vi "Mutate New CMD.vi"(0 "Class Library in":refnum<vi>, 1 "Line 2 text":string, 2 "Line 1 text":string, 5 "Command name":string, 7 "Wait For Response?":bool, 9 "Timeout":i32, 11 "error in":errorcluster) -> (4 "Class Library out":refnum<vi>, 15 "error out":errorcluster)   [LabVIEW 2012, in "REx_Springboard.lvlib"]
uses:
  REx_Springboard.lvlib
  <vilib>/LabVIEW Icon API/API_Text.ctl
  <vilib>/LabVIEW Icon API/API_Test Settings.ctl
  <vilib>/LabVIEW Icon API/lv_icon/Controls/Alignment.ctl
  <vilib>/LabVIEW Icon API/API_Text Colors.ctl
  <vilib>/LabVIEW Icon API/LabVIEW Icon API.lvlib
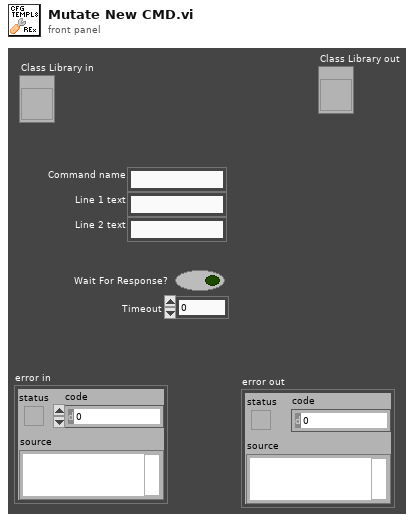
[diagram p1: front panel]
types:
  T1 = typedef "LabVIEW Icon API.lvlib/API_Text.ctl" = cluster{"Line 1 text":string, "Line 2 text":string, "Line 3 text":string, "Line 4 text":string}
  T2 = typedef "LabVIEW Icon API.lvlib/API_Test Settings.ctl" = cluster{"Font":string, "Alignment":T3, "Size":u8, "Center text":bool, "Capitalize text":bool, "Text color":T4}
  T3 = typedef "Alignment.ctl" = u16
  T4 = typedef "LabVIEW Icon API.lvlib/API_Text Colors.ctl" = cluster{"Line 1 color":u32, "Line 2 color":u32, "Line 3 color":u32, "Line 4 color":u32}
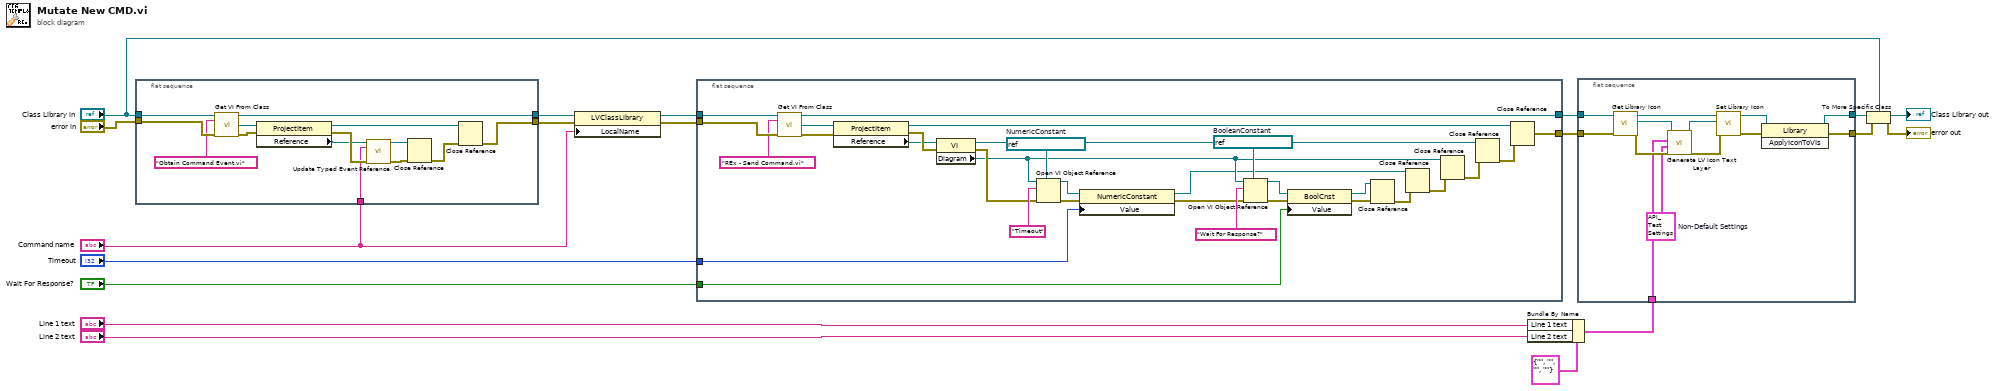
[diagram p0: block diagram]
diagram:
  n1 = flat-sequence {
    tunnel: [w27] -> w10
    tunnel: "Class Library in" -> [w26]
    tunnel: "error in" -> [w25]
    tunnel: [w20] -> w12
    tunnel: "Command name" -> [w23]
    frame #0 {
      n2 = call "Get VI From Class.vi"("Class Library"=w26, "Class Item Name"="Obtain Command Event.vi" ("Current Name 3"), "error in"=w25) -> ("Class Library"=w27:refnum<vi>, "Class Item Refnum"=w32:refnum<vi>, "error out"=w28:errorcluster)  [unwired: 10 in]
      n3 = property class="ProjectItem"(reference=w32, error in=w28) -> (reference out=w22:refnum<vi>, error out=w33:errorcluster, "Reference"=w31:refnum<vi>)
      n4 = call "Update Typed Event Reference.vi"("vi reference in"=w31, "Command Name"=w23, "error in"=w33) -> ("vi reference out"=w30:refnum<vi>, "error out"=w29:errorcluster)  [unwired: 11 in]
      n5 = Close Reference(reference=w30, error in (no error)=w29) -> (error out=w21:errorcluster)
      n6 = Close Reference(reference=w22, error in (no error)=w21) -> (error out=w20:errorcluster)
    }
  }
  n7 = property class="LVClassLibrary"(reference=w10, error in=w12, "LocalName"="Command name") -> (reference out=w13:refnum<vi>, error out=w15:errorcluster)
  n8 = flat-sequence {
    tunnel: "Wait For Response?" -> [w56]
    tunnel: [w34] -> w9
    tunnel: w13 -> [w55]
    tunnel: [w54] -> w14
    tunnel: w15 -> [w52]
    tunnel: "Timeout" -> [w49]
    frame #0 {
      w59 = refnum<vi> refnum  # BooleanConstant
      w61 = refnum<vi> refnum  # NumericConstant
      n9 = call "Get VI From Class.vi"("Class Library"=w55, "Class Item Name"="REx - Send Command.vi" ("name/order"), "error in"=w52) -> ("Class Library"=w54:refnum<vi>, "Class Item Refnum"=w53:refnum<vi>, "error out"=w46:errorcluster)  [unwired: 10 in]
      n10 = property class="ProjectItem"(reference=w53, error in=w46) -> (reference out=w44:refnum<vi>, error out=w64:errorcluster, "Reference"=w63:refnum<vi>)
      n11 = property class="VI"(reference=w63, error in=w64) -> (reference out=w43:refnum<vi>, error out=w50:errorcluster, "Diagram"=w42:refnum<vi>)
      n12 = Open VI Object Reference(7:w61, 8:w50, 10:"Timeout" ("name/order"), 11:w42) -> (0:w62:errorcluster, 3:w45:refnum<vi>)
      n13 = property class="NumericConstant"(reference=w45, error in=w62, "Value"=w49) -> (reference out=w41:refnum<vi>, error out=w48:errorcluster)
      n14 = Open VI Object Reference(7:w59, 8:w48, 10:"Wait For Response?" ("name/order"), 11:w42) -> (0:w47:errorcluster, 3:w58:refnum<vi>)
      n15 = property class="BoolCnst"(reference=w58, error in=w47, "Value"=w56) -> (reference out=w40:refnum<vi>, error out=w39:errorcluster)
      n16 = Close Reference(reference=w40, error in (no error)=w39) -> (error out=w38:errorcluster)
      n17 = Close Reference(reference=w41, error in (no error)=w38) -> (error out=w37:errorcluster)
      n18 = Close Reference(reference=w42, error in (no error)=w37) -> (error out=w36:errorcluster)
      n19 = Close Reference(reference=w43, error in (no error)=w36) -> (error out=w35:errorcluster)
      n20 = Close Reference(reference=w44, error in (no error)=w35) -> (error out=w34:errorcluster)
    }
  }
  n21 = Bundle By Name(cluster=T1 {"Line 1 text"="", "Line 2 text"="", "Line 3 text"="", "Line 4 text"=""} ("Text"), "Line 1 text"="Line 1 text", "Line 2 text"="Line 2 text") -> (w7:T1)
  n22 = flat-sequence {
    tunnel: w7 -> [w69]
    tunnel: [w65] -> w4
    tunnel: [w67] -> w6
    tunnel: w9 -> [w77]
    tunnel: w14 -> [w76]
    frame #0 {
      w68 = T2 {"Font"="Small Fonts", "Alignment"=1, "Size"=8, "Center text"=FALSE, "Capitalize text"=TRUE, "Text color"={"Line 1 color"=0, "Line 2 color"=0, "Line 3 color"=0, "Line 4 color"=0}}  # Non-Default Settings
      n23 = call <vilib>:"Get Library Icon.vi"("error in (no error)"=w77, "Library Refnum in"=w76) -> ("error out"=w72:errorcluster, "Icon"=w71:refnum<class "Icon.lvclass">, "Library Refnum out"=w73:refnum<vi>)  [unwired: 7 in]
      n24 = call <vilib>:"Generate LV Icon Text Layer.vi"("error in (no error)"=w72, "Text settings"=w68, "Text"=w69, "Icon in"=w71) -> ("error out"=w75:errorcluster, "Icon out"=w70:refnum<class "Icon.lvclass">)  [unwired: 6 in]
      n25 = call <vilib>:"Set Library Icon.vi"("error in (no error)"=w75, "Icon"=w70, "Library Refnum in"=w73) -> ("error out"=w74:errorcluster, "Library Refnum out"=w66:refnum<vi>)  [unwired: 7 in]
      n26 = invoke class="Library" method="ApplyIconToVIs"(reference=w66, error in=w74) -> (reference out=w65:refnum<vi>, error out=w67:errorcluster)  [unwired: 1 in, 1 out]
    }
  }
  n27 = To More Specific Class(target class="Class Library in", reference=w4, error in=w6) -> (specific class reference=→"Class Library out":refnum<vi>, error out=→"error out":errorcluster)
